vi "Configure 4-port Network (De-)Embedding.vi"(0 "VISA resource name":refnum<visa-resource-name>, 1 "Network Type (0: No-processing)":u16(ring) items=["No-processing", "Embedding", "De-embedding"], 2 "Network (1)":i32=1, 3 "Port 1 (1)":i32=1, 4 "Port 2 (2)":i32=2, 5 "error in (no error)":errorcluster, 6 "Channel (1)":i32=1, 7 "Port 3 (3)":i32=3, 8 "Topology Type (0: A)":u16(ring) items=["A", "B", "C"], 9 "Port 4 (4)":i32=4, 10 "Network Embedding/De-embeding State (F: Disable)":bool, 13 "Network File (\"\")":string) -> (14 "VISA resource name out":refnum<visa-resource-name>, 19 "error out":errorcluster)   [LabVIEW 2020, in "Agilent ENA Series.lvlib"]
doc: "Configures 4-port network embedding/de-embedding.\n\nNotes:\nThis function is available with the firmware version 3.50 or greater.\nThis VI is not supported by the E5063A model."
uses:
  <instrlib>/Agilent ENA Series/Agilent ENA Series.lvlib
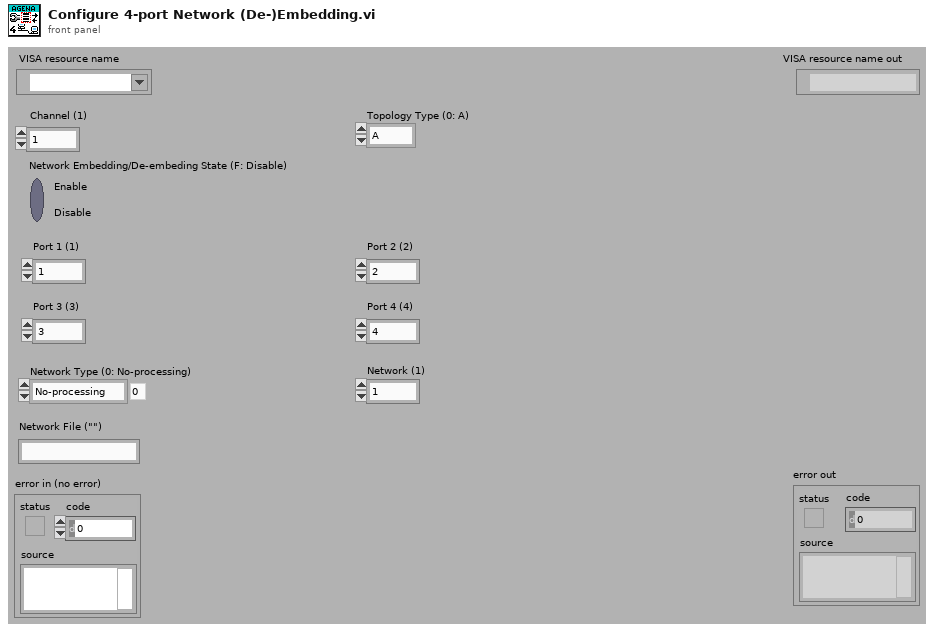
[diagram p1: front panel]
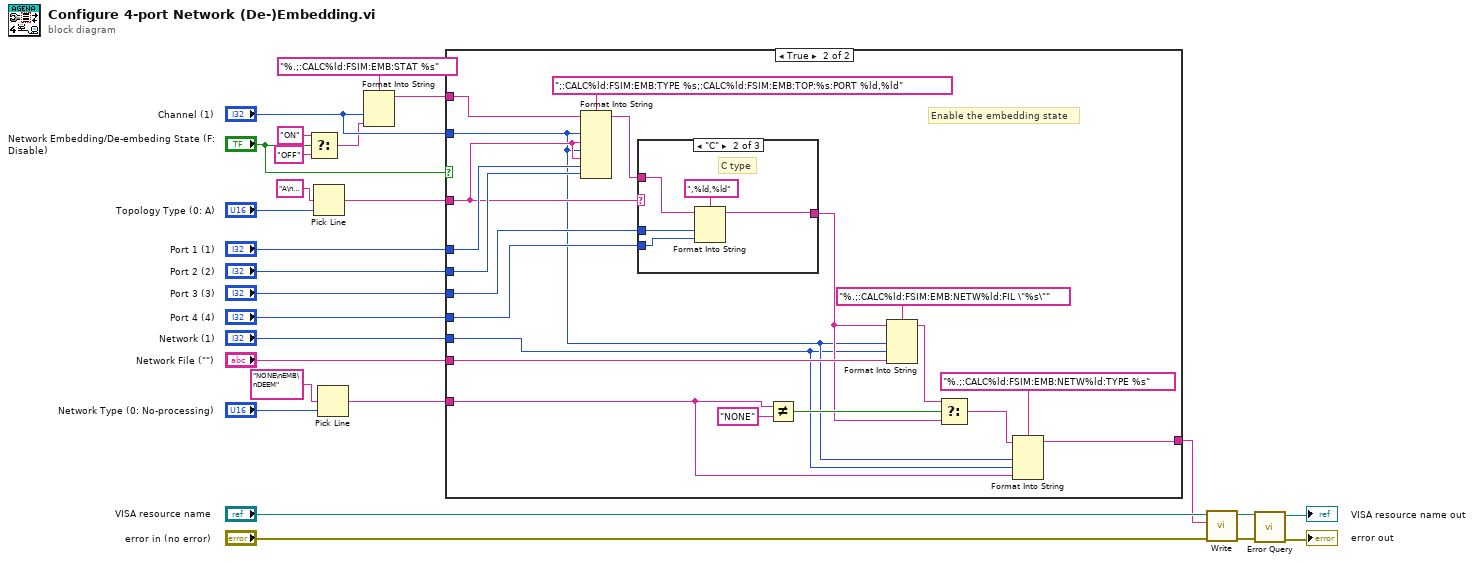
[diagram p0: block diagram]
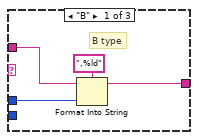
[diagram p3: hidden frame]
diagram:
  n1 = Select(t="ON", s="Network Embedding/De-embeding State (F: Disable)", f="OFF") -> (s? t:f=w16:string)
  n2 = Pick Line(multi-line string="A\nB\nC", line index="Topology Type (0: A)") -> (output string=w11:string)  [unwired: 1 in]
  n3 = Pick Line(multi-line string="NONE\nEMB\nDEEM", line index="Network Type (0: No-processing)") -> (output string=w6:string)  [unwired: 1 in]
  n4 = Format Into String(format string="%.;:CALC%ld:FSIM:EMB:STAT %s", "Channel (1)", w16) -> (resulting string=w14:string)  [unwired: 2 in, 1 out]
  n5 = case shown="True" "Network Embedding/De-embeding State (F: Disable)" {
    tunnel: "Channel (1)" -> [_ w32]
    tunnel: "Network File (\"\")" -> [_ w36]
    tunnel: [w27 w28] -> w15
    tunnel: w14 -> [w27 w44]
    tunnel: w11 -> [_ w41]
    tunnel: "Port 1 (1)" -> [_ w43]
    tunnel: "Port 2 (2)" -> [_ w42]
    tunnel: "Port 3 (3)" -> [_ w40]
    tunnel: "Port 4 (4)" -> [_ w38]
    tunnel: w6 -> [_ w30]
    tunnel: "Network (1)" -> [_ w31]
    frame False {
      # "Disable the embedding state"
    }
    frame True {
      # "Enable the embedding state"
      n6 = Format Into String(format string=";:CALC%ld:FSIM:EMB:TYPE %s;:CALC%ld:FSIM:EMB:TOP:%s:PORT %ld,%ld", initial string=w44, w32, w41, w32, w41, w43, w42) -> (resulting string=w39:string)  [unwired: 1 in, 1 out]
      n7 = case shown="\"C\"" w41 {
        tunnel: w40 -> [w50 w55 _]
        tunnel: w39 -> [w49 w53 w57]
        tunnel: [w48 w52 w57] -> w34
        tunnel: w38 -> [_ w54 _]
        frame "B" {
          # "B type"
          n8 = Format Into String(format string=",%ld", initial string=w49, w50) -> (resulting string=w48:string)  [unwired: 1 in, 1 out]
        }
        frame "C" {
          # "C type"
          n9 = Format Into String(format string=",%ld,%ld", initial string=w53, w55, w54) -> (resulting string=w52:string)  [unwired: 1 in, 1 out]
        }
        frame "A", Default {
          # "A type"
        }
      }
      n10 = Not Equal?(x=w30, y="NONE") -> (x != y?=w45:bool)
      n11 = Format Into String(format string="%.;:CALC%ld:FSIM:EMB:NETW%ld:FIL \"%s\"", initial string=w34, w32, w31, w36) -> (resulting string=w35:string)  [unwired: 1 in, 1 out]
      n12 = Select(t=w35, s=w45, f=w34) -> (s? t:f=w29:string)
      n13 = Format Into String(format string="%.;:CALC%ld:FSIM:EMB:NETW%ld:TYPE %s", initial string=w29, w32, w31, w30) -> (resulting string=w28:string)  [unwired: 1 in, 1 out]
    }
  }
  n14 = call <instrlib>:"Write.vi"("error in (no error)"="error in (no error)", "String ()"=w15, "VISA resource name"="VISA resource name") -> ("error out"=w3:errorcluster, "VISA resource name out"=w4:refnum<visa-resource-name>)  [unwired: 6 in, 1 out]
  n15 = call <instrlib>:"Error Query.vi"("error in (no error)"=w3, "VISA resource name"=w4) -> ("error out"=→"error out":errorcluster, "VISA resource name out"=→"VISA resource name out":refnum<visa-resource-name>)  [unwired: 6 in, 2 out]
